vi "MainWindow.vi"() -> ()   [LabVIEW 2017]
doc: "Main Window. This VI handles the constant readout of the SystemDevices (Gauges, Temp,... NOT the switches)"
uses:
  global variables.vi
  Classes/Message/Message.lvclass
panel:
  out "message string":string
  # "MS Control"
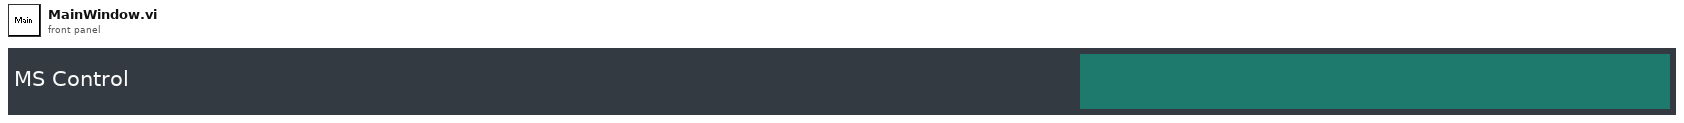
[diagram p1: front panel]
types:
  T1 = typedef "LVRectTypeDef.ctl" = cluster{"Left":i16, "Top":i16, "Right":i16, "Bottom":i16}
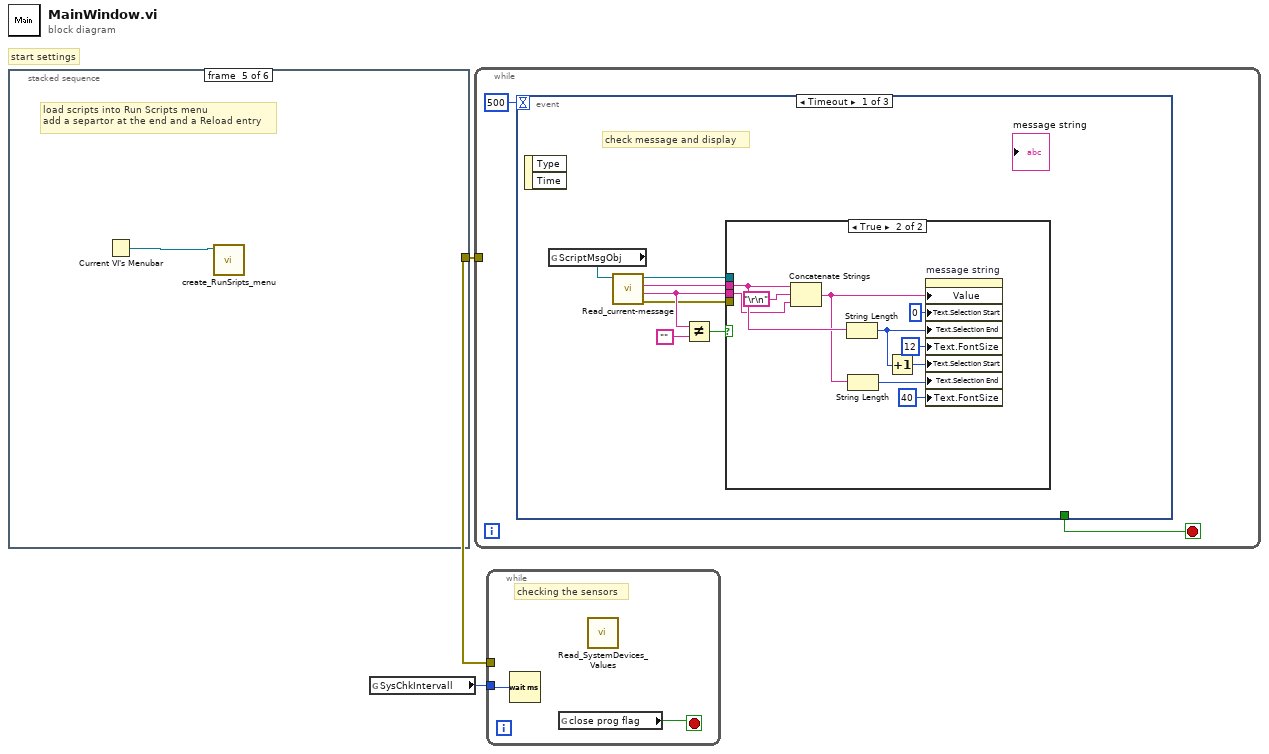
[diagram p0: block diagram]
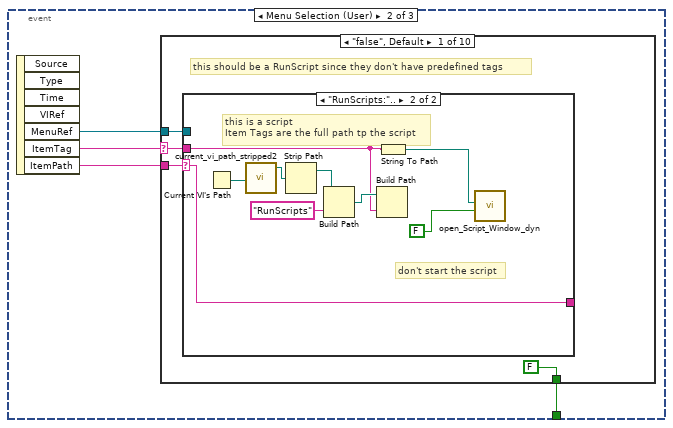
[diagram p3: hidden frame]
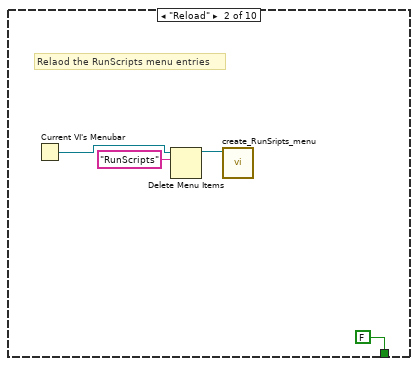
[diagram p5: hidden frame]
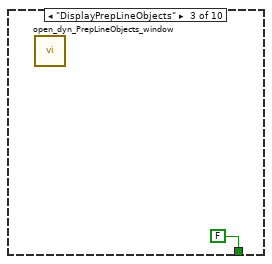
[diagram p6: hidden frame]
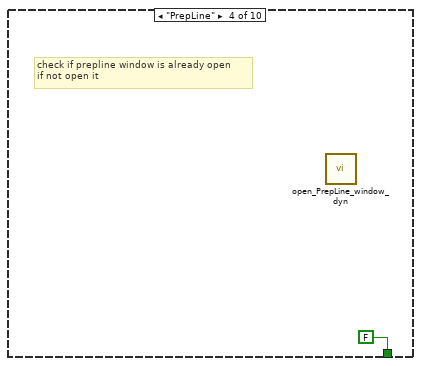
[diagram p7: hidden frame]
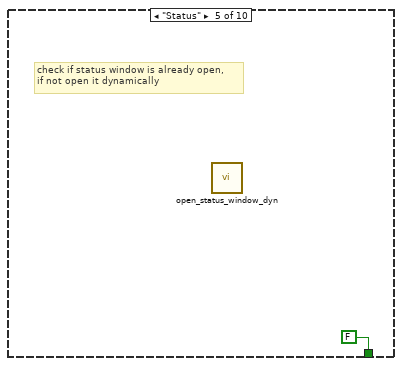
[diagram p8: hidden frame]
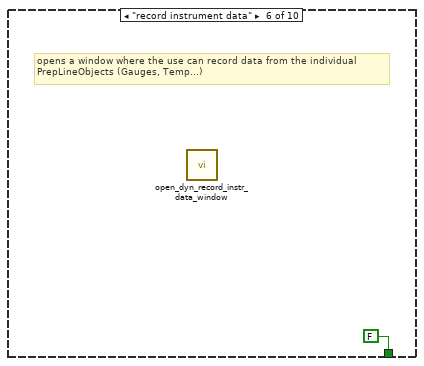
[diagram p9: hidden frame]
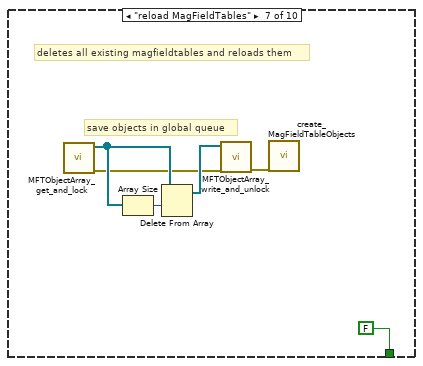
[diagram p10: hidden frame]
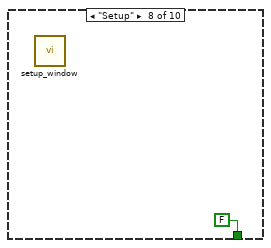
[diagram p11: hidden frame]
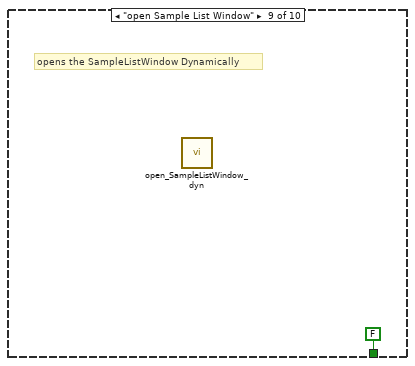
[diagram p12: hidden frame]
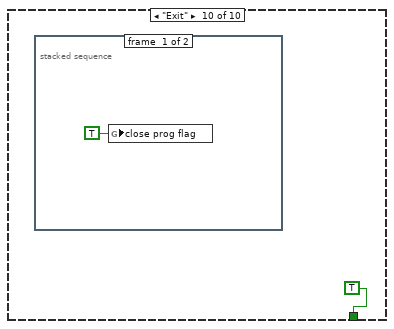
[diagram p13: hidden frame]
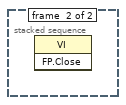
[diagram p14: hidden frame]
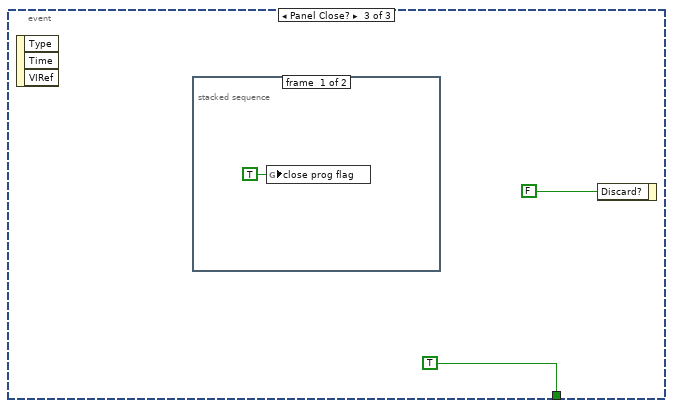
[diagram p15: hidden frame]
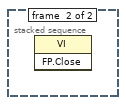
[diagram p16: hidden frame]
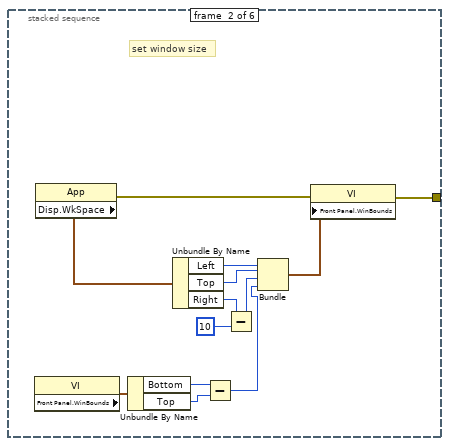
[diagram p18: hidden frame]
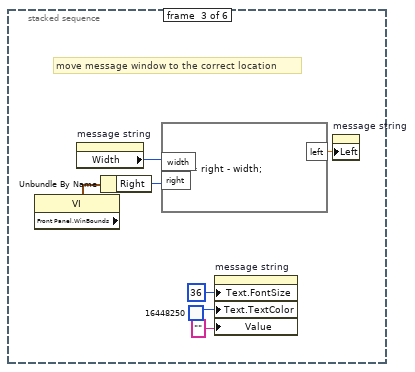
[diagram p19: hidden frame]
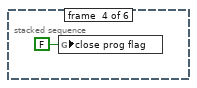
[diagram p20: hidden frame]
diagram:
  # "start settings"
  n1 = stacked-sequence {
    tunnel: [_ w7 _ _ _ _] -> w2
    frame #0 {
      # "obtain global Queues again in order to keep them in memory\nfor the duration of the run-time"
    }
    frame #1 {
      # "set window size"
      n2 = property class="VI"() -> ("Front Panel.WinBounds"=w6:T1)  [unwired: 2 in, 2 out]
      n3 = property class="App"() -> (error out=w8:errorcluster, "Disp.WkSpace"=w15:T1)  [unwired: 2 in, 1 out]
      n4 = Unbundle By Name(w6) -> ("Bottom"=w5:i16, "Top"=w4:i16)
      n5 = Unbundle By Name(w15) -> ("Left"=w14:i16, "Top"=w13:i16, "Right"=w11:i16)
      n6 = Subtract(x=w5, y=w4) -> (x-y=w3:i16)
      n7 = Subtract(x=w11, y=i16 10) -> (x-y=w9:i16)
      n8 = Bundle("Left"=w14, "Top"=w13, w9, w3) -> (w12:cluster{"Left":i16, "Top":i16, i16, i16})  [unwired: 1 in]
      n9 = property class="VI"(error in=w8, "Front Panel.WinBounds"=w12) -> (error out=w7:errorcluster)  [unwired: 1 in, 1 out]
    }
    frame #2 {
      # "move message window to the correct location"
      n10 = property class="VI"() -> ("Front Panel.WinBounds"=w22:T1)  [unwired: 2 in, 2 out]
      n11 = property on="message string" class="Str"() -> ("Width"=w21:u32)  [unwired: 2 in, 2 out]
      n12 = Unbundle By Name(w22) -> ("Right"=w20:i16)
      n13 = formula code="left = right - width;"("width"=w21, "right"=w20) -> ("left"=w19:dbl)
      n14 = property on="message string" class="Str"("Text.FontSize"=u32 36 ("Text.Font:Size"), "Text.TextColor"=u32 16448250, "Value"="" ("message string")) -> ()  [unwired: 2 in, 2 out]
      n15 = property on="message string" class="Str"("Left"=w19) -> ()  [unwired: 2 in, 2 out]
    }
    frame #3 {
      n16 = global write "global variables.vi" "close prog flag"(FALSE ("close prog flag")) -> ()
    }
    frame #4 {
      # "load scripts into Run Scripts menu\nadd a separtor at the end and a Reload entry"
      n17 = Current VI's Menubar() -> (w24:refnum<k9>)
      n18 = call "create_RunSripts_menu.vi"("menu reference"=w24) -> ()  [unwired: 11 in]
    }
    frame #5 {
      n19 = Wait (ms)(milliseconds to wait=u32 2000) -> ()  [unwired: 1 out]
    }
  }
  n20 = global read "global variables.vi" "SysChkIntervall"() -> (w1:u32)
  n21 = while {
    tunnel: w2 -> [_]
    stop <- w27 stop-if-true
    n22 = event shown="[0] Timeout" {
      selector: _ -> [_ _ _]
      dyn-events: _ -> [_ _ _]
      timeout: 500 -> [_ _ _]
      tunnel: [_ w46 TRUE] -> w27
      event Timeout {
        # "check message and display"
        n23 = event-data() -> ()  [unwired: 1 in, 2 out]
        n24 = global read "global variables.vi" "ScriptMsgObj"() -> (w32:refnum<class "Message.lvclass">)
        n25 = call-dynamic "Read_current-message.vi"("Message in"=w32) -> ("error out"=w28:errorcluster, "message string"=w30:string, "time string"=w31:string, "Message out"=w29:refnum<class "Message.lvclass">)  [unwired: 6 in, 1 out]
        n26 = Not Equal?(x=w30, y="") -> (x != y?=w34:bool)
        n27 = case shown="True" w34 {
          tunnel: w31 -> [_ w44]
          tunnel: w30 -> [_ w42]
          tunnel: w29 -> [_ _]
          tunnel: w28 -> [_ _]
          frame False {
          }
          frame True {
            n28 = Concatenate Strings(w44, "\r\n", w42) -> (w39:string)
            n29 = String Length(string=w44) -> (length=w38:i32)
            n30 = String Length(string=w39) -> (length=w36:i32)
            n31 = Increment(x=w38) -> (x+1=w37:i32)
            n32 = property on="message string" class="Str"("Value"=w39, "Text.Selection Start"=u32 0 ("Text.Selection:Start"), "Text.Selection End"=w38, "Text.FontSize"=u32 12 ("Text.Font:Size"), "Text.Selection Start"=w37, "Text.Selection End"=w36, "Text.FontSize"=u32 40 ("Text.Font:Size")) -> ()  [unwired: 2 in, 2 out]
          }
        }
      }
      event Menu Selection (User) {
        n33 = event-data() -> ("MenuRef"=w45:refnum<k9>, "ItemTag"=w48:string, "ItemPath"=w47:string)  [unwired: 1 in, 4 out]
        n34 = case shown="\"false\", Default" w48 {
          selector: w48 -> [w51 _ _ _ _ _ _ _ _ _]
          tunnel: w47 -> [w52 _ _ _ _ _ _ _ _ _]
          tunnel: [FALSE FALSE FALSE FALSE FALSE FALSE FALSE FALSE FALSE TRUE] -> w46
          tunnel: w45 -> [w49 _ _ _ _ _ _ _ _ _]
          frame "false", Default {
            # "this should be a RunScript since they don't have predefined tags"
            n35 = case shown="\"RunScripts:\".." w52 {
              selector: w52 -> [_ w55]
              tunnel: w51 -> [_ w53]
              tunnel: w49 -> [_ _]
              tunnel: [_ w55] -> _
              frame "False", Default {
              }
              frame "RunScripts:".. {
                # "don't start the script"
                # "this is a script\nItem Tags are the full path tp the script"
                n36 = Current VI's Path() -> (path=w58:path)
                n37 = call "current_vi_path_stripped2.vi"("current VI Path"=w58) -> ("current VI Path stripped out"=w57:path)  [unwired: 3 in, 1 out]
                n38 = Strip Path(path=w57) -> (stripped path=w56:path)  [unwired: 1 out]
                n39 = Build Path(base path=w56, name or relative path="RunScripts") -> (appended path=w60:path)
                n40 = Build Path(base path=w60, name or relative path=w53) -> ()  [unwired: 1 out]
                n41 = String To Path(string=w53) -> (path=w54:path)
                n42 = call "open_Script_Window_dyn.vi"("run/stop button"=FALSE, "Script Path"=w54) -> ()  [unwired: 9 in, 1 out]
              }
            }
          }
          frame "Reload" {
            # "Relaod the RunScripts menu entries"
            n43 = Current VI's Menubar() -> (w63:refnum<k9>)
            n44 = Delete Menu Items(8:"RunScripts" ("menu tag"), 9:w63) -> (3:w62:refnum<k9>)  [unwired: 2 in, 1 out]
            n45 = call "create_RunSripts_menu.vi"("menu reference"=w62) -> ()  [unwired: 11 in]
          }
          frame "DisplayPrepLineObjects" {
            n46 = call "open_dyn_PrepLineObjects_window.vi"() -> ()  [unwired: 11 in, 1 out]
          }
          frame "PrepLine" {
            # "check if prepline window is already open\nif not open it"
            n47 = call "open_PrepLine_window_dyn.vi"() -> ()  [unwired: 11 in, 1 out]
          }
          frame "Status" {
            # "check if status window is already open,\nif not open it dynamically"
            n48 = call "open_status_window_dyn.vi"() -> ()  [unwired: 11 in, 1 out]
          }
          frame "record instrument data" {
            # "opens a window where the use can record data from the individual\nPrepLineObjects (Gauges, Temp...)"
            n49 = call "open_dyn_record_instr_data_window.vi"() -> ()  [unwired: 11 in, 1 out]
          }
          frame "reload MagFieldTables" {
            # "save objects in global queue"
            # "deletes all existing magfieldtables and reloads them"
            n50 = call "MFTObjectArray_get_and_lock.vi"() -> ("error out"=w72:errorcluster, "MFTObjects"=w75:refnum<class "MagFieldTable.lvclass">[])  [unwired: 10 in]
            n51 = Array Size(array=w75) -> (size(s)=w74:i32)
            n52 = Delete From Array(array=w75, length=w74) -> (array with subset deleted=w73:refnum<class "MagFieldTable.lvclass">[])  [unwired: 1 in, 1 out]
            n53 = call "MFTObjectArray_write_and_unlock.vi"("error in (no error)"=w72, "MFTObjects"=w73) -> ("error out"=w71:errorcluster)  [unwired: 9 in]
            n54 = call "create_MagFieldTableObjects.vi"("error in (no error)"=w71) -> ()  [unwired: 10 in, 1 out]
          }
          frame "Setup" {
            n55 = call "setup_window.vi"() -> ()  [unwired: 12 in]
          }
          frame "open Sample List Window" {
            # "opens the SampleListWindow Dynamically"
            n56 = call "open_SampleListWindow_dyn.vi"() -> ()  [unwired: 11 in, 1 out]
          }
          frame "Exit" {
            n57 = stacked-sequence {
              frame #0 {
                n58 = global write "global variables.vi" "close prog flag"(TRUE ("close prog flag")) -> ()
              }
              frame #1 {
                n59 = invoke class="VI" method="FP.Close"() -> ()  [unwired: 3 in, 3 out]
              }
            }
          }
        }
      }
      event Panel Close? {
        n60 = event-data() -> ()  [unwired: 1 in, 3 out]
        n61 = stacked-sequence {
          frame #0 {
            n62 = global write "global variables.vi" "close prog flag"(TRUE ("close prog flag")) -> ()
          }
          frame #1 {
            n63 = invoke class="VI" method="FP.Close"() -> ()  [unwired: 3 in, 3 out]
          }
        }
        n64 = event-data("Discard?"=FALSE) -> ()  [unwired: 1 in, 1 out]
      }
    }
  }
  n65 = while {
    tunnel: w2 -> [_]
    tunnel: w1 -> [w83]
    stop <- w84 stop-if-true
    # "checking the sensors"
    n66 = Wait (ms)(milliseconds to wait=w83) -> ()  [unwired: 1 out]
    n67 = global read "global variables.vi" "close prog flag"() -> (w84:bool)
    n68 = call "Read_SystemDevices_Values.vi"() -> ()  [unwired: 11 in, 1 out]
  }
